vi "Main.vi"() -> ()   [LabVIEW 2021]
doc: "This template is for the Queued Message Handler design pattern.\n\nThe Event Handling Loop generates messages based on user interface actions.\n\nThe Message Handling Loop processes messages generated by the Event Handling Loop, or by other messages. The messages are string values, so new messages can be added easily to the Message Cases case structure in the Message Handling Loop. Each message cluster can also provide an optional value for Message Data, which is a variant that can be converted to whatever message-specific data is required."
uses:
  controls/Air SAS Controls.ctl
  <vilib>/MakerHub/LINX/Private/Type Defs/LINX Ref.ctl
  <vilib>/MakerHub/LINX/Private/Type Defs/Platform.ctl
  <vilib>/MakerHub/LINX/Private/Type Defs/Interface.ctl
  <vilib>/MakerHub/LINX/Private/Device/Type Defs/LINX Device Config.ctl
  <vilib>/MakerHub/LINX/Private/Device/Type Defs/TCP Config.ctl
  <vilib>/MakerHub/LINX/Private/Device/Type Defs/Channels.ctl
  support/Message Queue/Enqueue Message (Single).vi
  <vilib>/MakerHub/LINX/Public/Utilities/Open Serial.vi
  <vilib>/Utility/error.llb/Error Cluster From Error Code.vi
  <vilib>/ErrorRing/Error Ring.xnode
  support/Message Queue/Message Queue.lvlib
  support/User Event - Stop/User Event - Stop.lvlib
  <vilib>/MakerHub/LINX/LMH-LINX.lvlib
  <vilib>/MakerHub/LINX/Private/Device/Device.lvlib
panel:
  in  "Motion Control":bool
  in  "Serial Port":refnum<visa-resource-name>="COM3"
  out "Display <Replace Me>":string
  in  "SAS Data Acquisition":bool
  in  "Waveform Capture":bool
  in  "Exit":bool
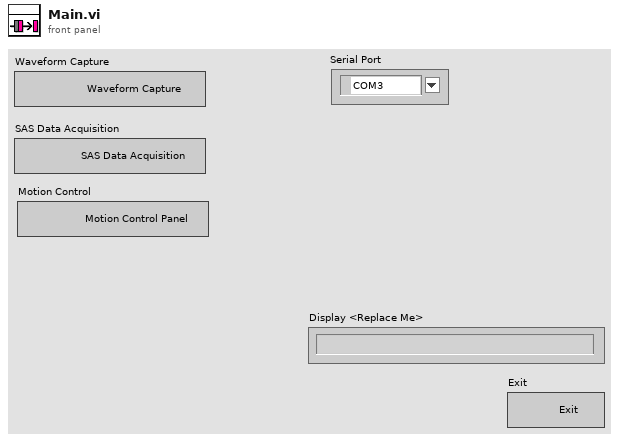
[diagram p1: front panel]
types:
  T1 = enum8{"Enabled", "Disabled", "Disabled and Grayed Out"}
  T2 = typedef "Air SAS Controls.ctl" = cluster{"Receive Duration":dbl, "I/O":cluster{"DAQmx Device":tag, "AO Range":dbl, "AI Range":dbl, "DAQ Group Delay":dbl, "Fs":dbl}, "Hardware":cluster{"Centerpos":dbl[], "TXpos":dbl[], "RX1pos":dbl[], "RX2pos":dbl[], "Angle":dbl, "Height":dbl}, "Waveform":cluster{"LFM Parameters":cluster{"Duration":dbl, "Fstart (Hz)":dbl, "Fstop (Hz)":dbl, "Out. Amplitude (Vpk)":dbl, "Window %":dbl}, "Transmit Waveform":waveform(dbl)}, "LINX Resource":T3, "Port":dbl}
  T3 = typedef "LMH-LINX.lvlib/LINX Ref.ctl" = cluster{"IO":T4, "Interface":T5, "LINX Device Config":T6}
  T4 = typedef "LMH-LINX.lvlib/Platform.ctl" = enum16{"Remote", "Local"}
  T5 = typedef "LMH-LINX.lvlib/Interface.ctl" = enum16{"Serial", "TCP"}
  T6 = typedef "LMH-LINX.lvlib/Device.lvlib/LINX Device Config.ctl" = cluster{"Interface":T5, "COM Port":refnum<visa-resource-name>, "TCP Configuration":T7, "Device Family":u8, "Device ID":u8, "Device Name":string, "TCP Ref":refnum<k5>, "Channels":T8}
  T7 = typedef "LMH-LINX.lvlib/Device.lvlib/TCP Config.ctl" = cluster{"IP Address":string, "Port":u16}
  T8 = typedef "LMH-LINX.lvlib/Channels.ctl" = cluster{"DI":u8[], "DO":u8[], "AI":u8[], "AO":u8[], "PWM":u8[], "QE":u8[], "UART":u8[], "I2C 2":u8[], "SPI":u8[], "CAN":u8[], "Servo":u8[], "AI Ref (V)":dbl, "AI Resolution (Bits)":u8, "AO Ref (V)":dbl, "AO Resolution (Bits)":u8}
  T9 = typedef "Message Queue.lvlib/All Message Queues.ctl" = cluster{"UI":refnum<queue>}
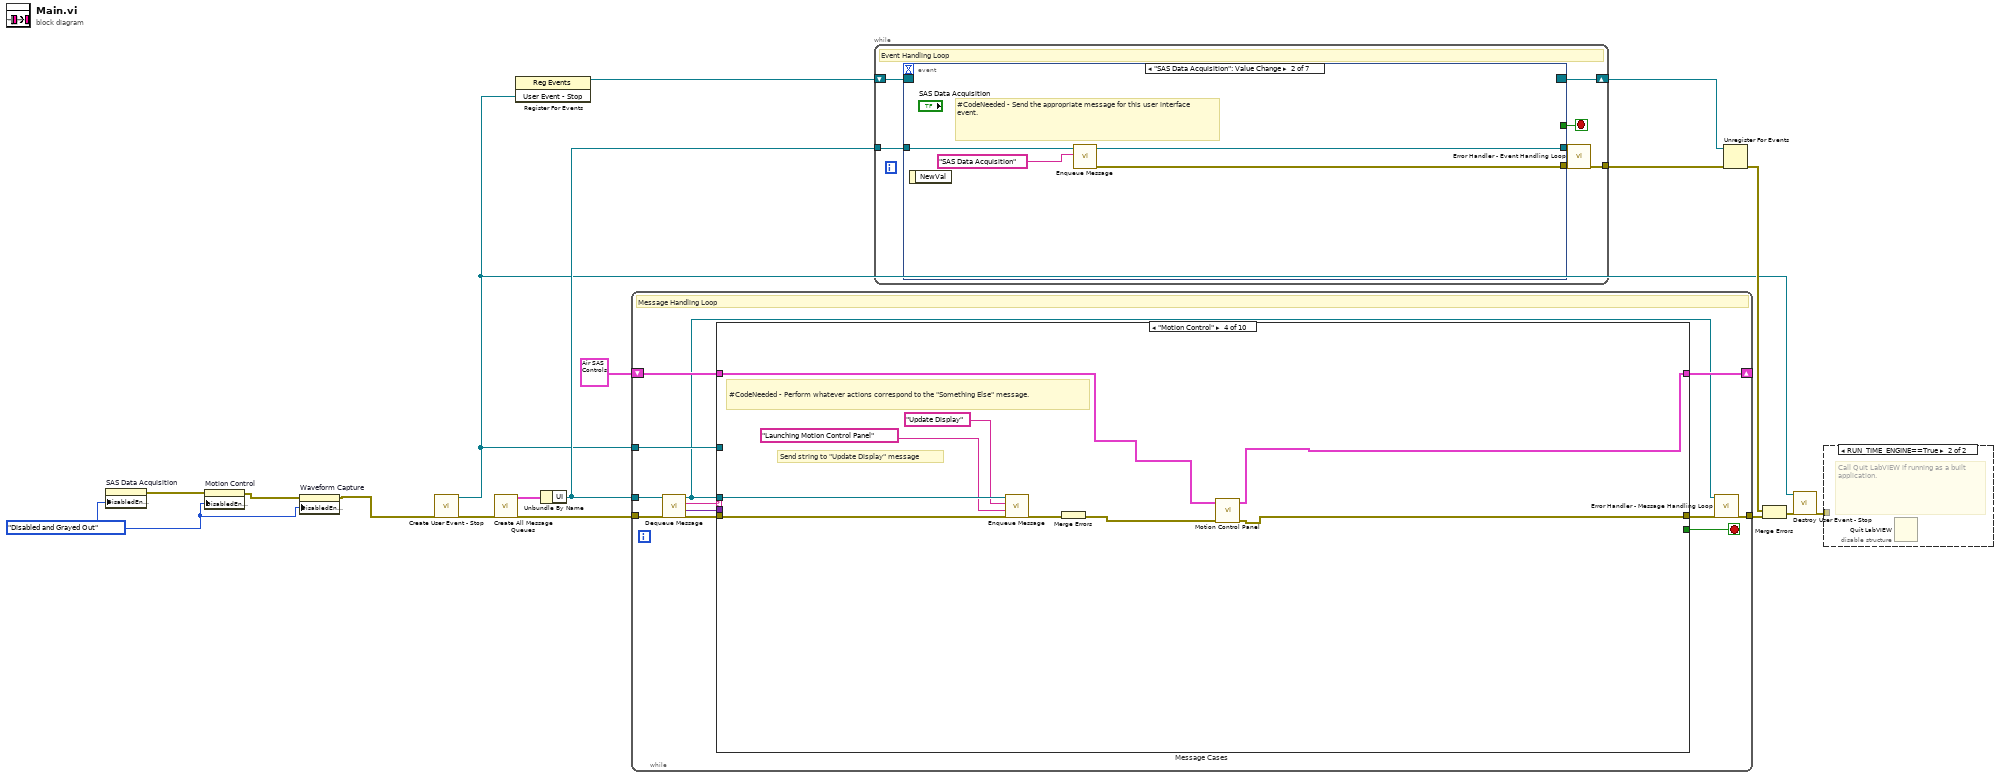
[diagram p0: block diagram]
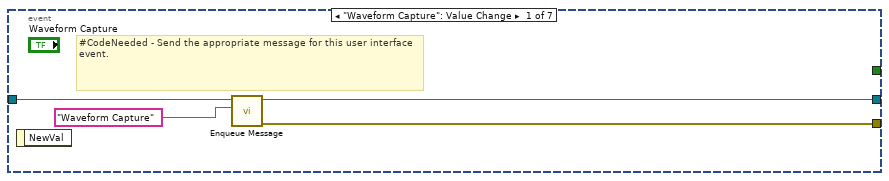
[diagram p3: hidden frame]
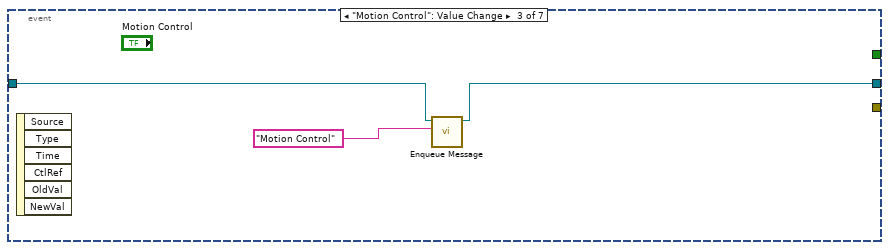
[diagram p4: hidden frame]
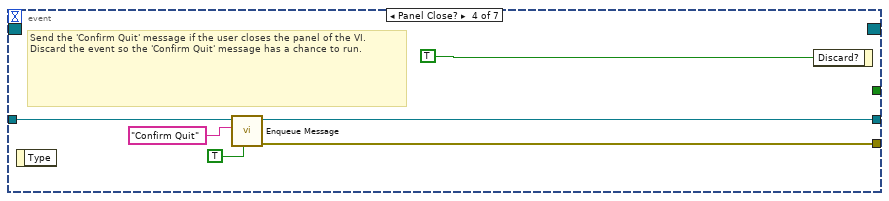
[diagram p5: hidden frame]
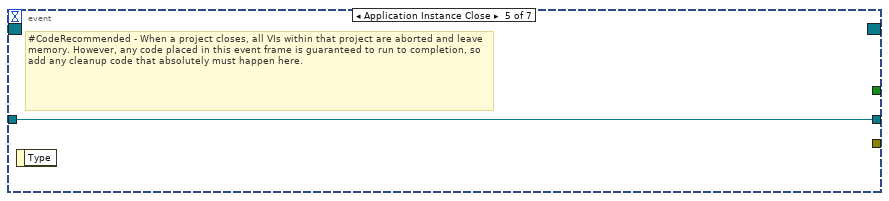
[diagram p6: hidden frame]
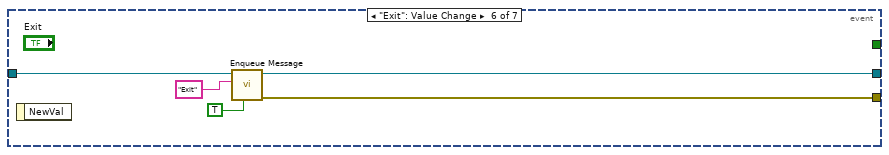
[diagram p7: hidden frame]
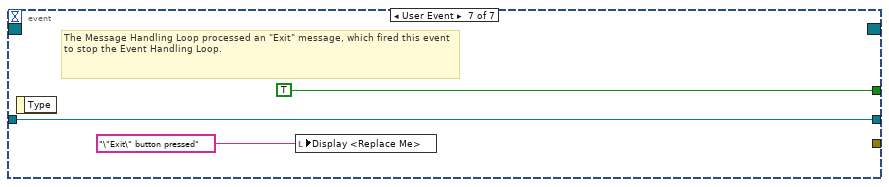
[diagram p8: hidden frame]
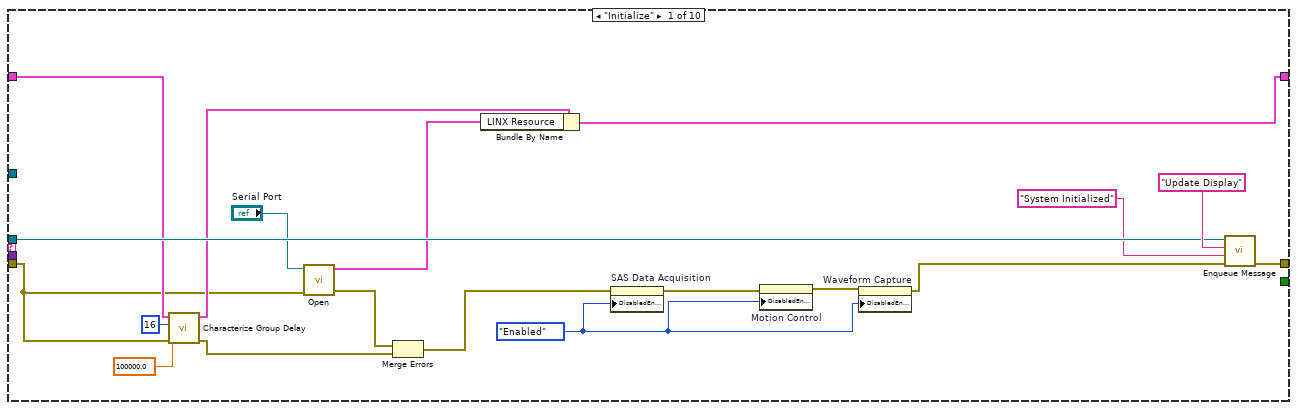
[diagram p9: hidden frame]
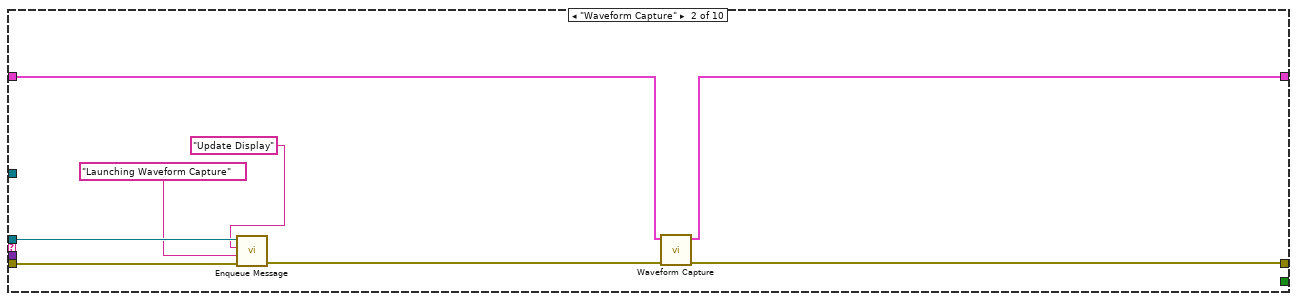
[diagram p10: hidden frame]
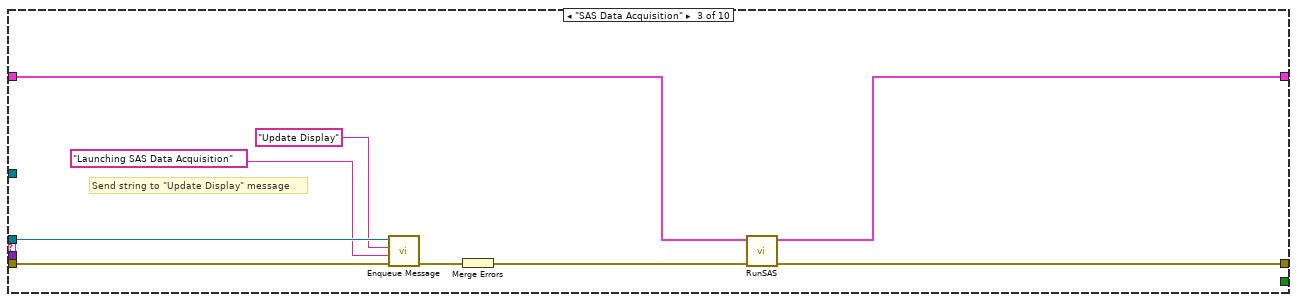
[diagram p11: hidden frame]
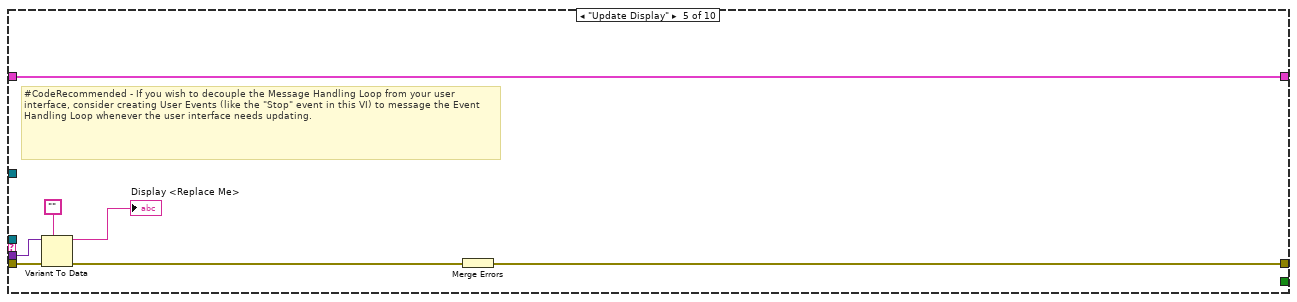
[diagram p12: hidden frame]
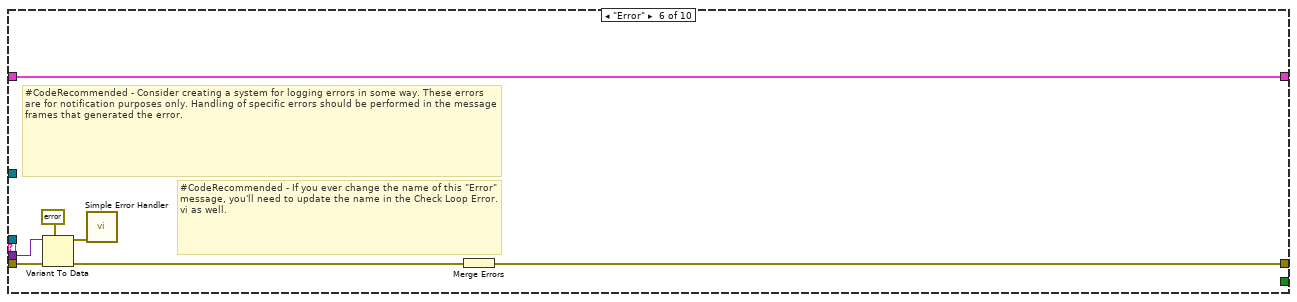
[diagram p13: hidden frame]
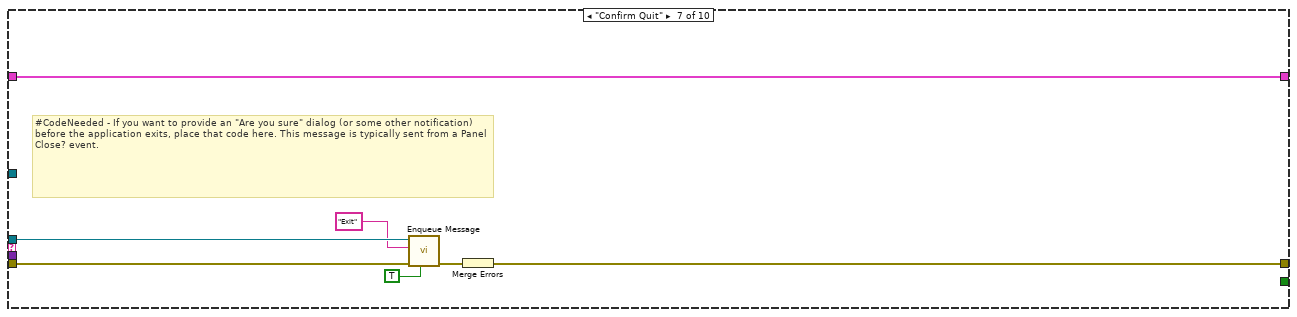
[diagram p14: hidden frame]
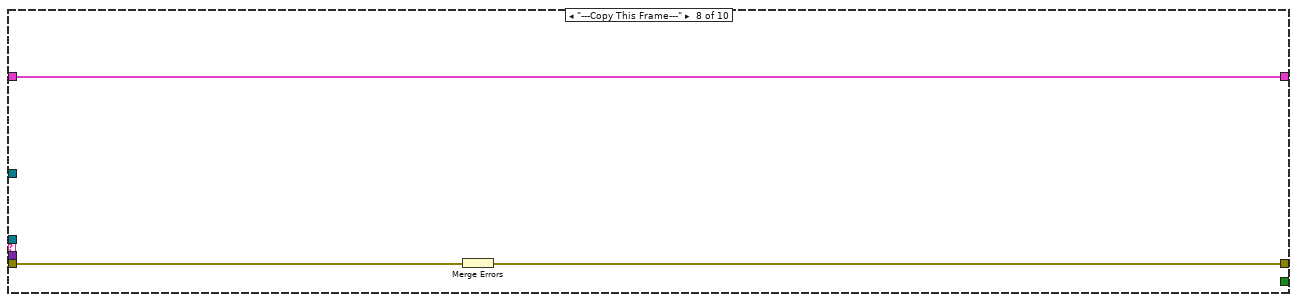
[diagram p15: hidden frame]
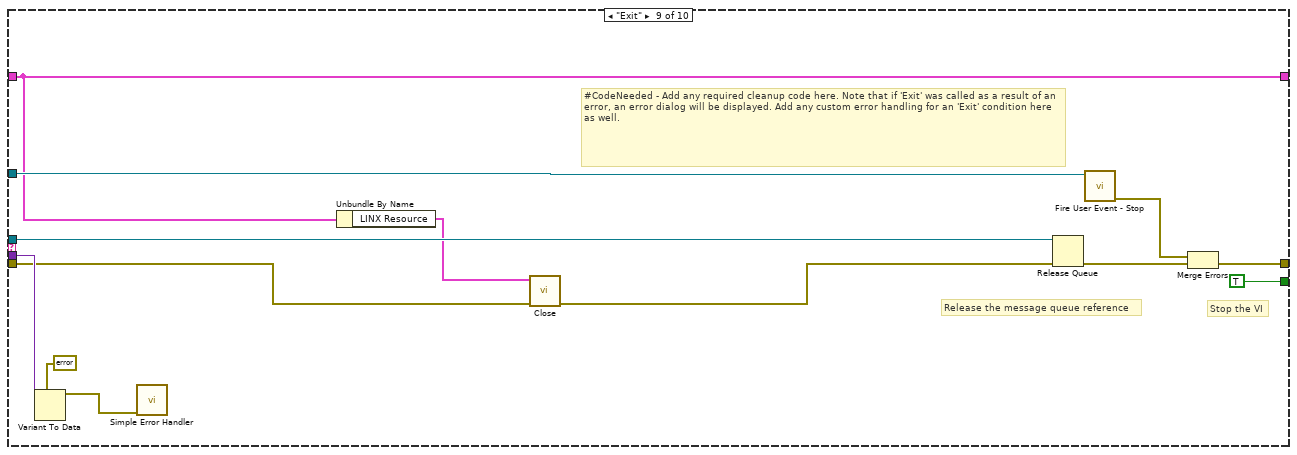
[diagram p16: hidden frame]
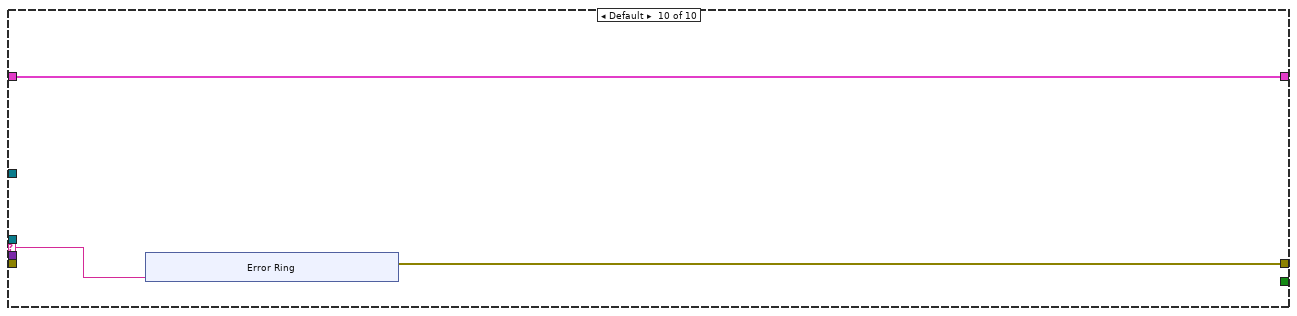
[diagram p17: hidden frame]
diagram:
  w1 = T1."Disabled and Grayed Out" ("Disabled")
  n1 = property on="SAS Data Acquisition" class="Bool"("DisabledEnum"=w1) -> (error out=w4:errorcluster)  [unwired: 2 in, 1 out]
  n2 = property on="Motion Control" class="Bool"(error in=w4, "DisabledEnum"=w1) -> (error out=w3:errorcluster)  [unwired: 1 in, 1 out]
  n3 = property on="Waveform Capture" class="Bool"(error in=w3, "DisabledEnum"=w1) -> (error out=w2:errorcluster)  [unwired: 1 in, 1 out]
  n4 = call "Create User Event - Stop.vi"("error in (no error)"=w2) -> ("error out"=w13:errorcluster, "User Event - Stop"=w6:refnum<user-event>)  [unwired: 9 in]
  n5 = call "Create All Message Queues.vi"("error in (no error)"=w13) -> ("error out"=w17:errorcluster, "Message Queues out"=w16:T9)  [unwired: 9 in]
  n6 = register-events(w6) -> (reference out=w7:refnum<event-registration>)  [unwired: 2 in, 1 out]
  n7 = Unbundle By Name(w16) -> ("UI"=w14:refnum<queue>)
  n8 = while {
    tunnel: w14 -> [w21]
    shift-right: [w28] -> _
    shift-left: T2 {"Receive Duration"=0.0, "I/O"={"DAQmx Device"="Dev1", "AO Range"=0.0, "AI Range"=0.0, "DAQ Group Delay"=0.0, "Fs"=0.0}, "Hardware"={"Centerpos"=[0.0, 0.0, 0.0], "TXpos"=[0.0, 0.0, 0.0], "RX1pos"=[0.0, 0.0, 0.0], "RX2pos"=[0.0, 0.0, 0.0], "Angle"=0.0, "Height"=0.0}, "Waveform"={"LFM Parameters"={"Duration"=1.0, "Fstart (Hz)"=1000.0, "Fstop (Hz)"=10000.0, "Out. Amplitude (Vpk)"=1.0, "Window %"=10.0}, "Transmit Waveform"={"t0"=timestamp(0 s since 1904-01-01), "dt"=1.0, "Y"=[]}}, "LINX Resource"={"IO"=enum."Remote", "Interface"=enum."Serial", "LINX Device Config"={"Interface"=enum."Serial", "COM Port"="COM13", "TCP Configuration"={"IP Address"="", "Port"=0}, "Device Family"=1, "Device ID"=1, "Device Name"="myRIO-1900", "TCP Ref"=refnum, "Channels"={"DI"=[0, 1, 2, 3, 4, 5, 6, 7, 8, 9, 10, 11, 12, 13, 14, 15, 16, 17, 18, 19, 20, 21, 22, 23, 24, 25, 26, 27, 28, 29, 30, 31, 32, 33, 34, 35, 36, 37, 38, 39, 40, 41, 42, 43, 44, 45, 46], "DO"=[0, 1, 2, 3, 4, 5, 6, 7, 8, 9, 10, 11, 12, 13, 14, 15, 16, 17, 18, 19, 20, 21, 22, 23, 24, 25, 26, 27, 28, 29, 30, 31, 32, 33, 34, 35, 36, 37, 38, 39, 40, 41, 42, 43, 44, 45, 46], "AI"=[0, 1, 2, 3, 4, 5, 6, 7, 8, 9, 10, 11], "AO"=[], "PWM"=[3, 5, 6, 9, 10], "QE"=[], "UART"=[0, 1], "I2C 2"=[0], "SPI"=[0], "CAN"=[], "Servo"=[], "AI Ref (V)"=0.0, "AI Resolution (Bits)"=0, "AO Ref (V)"=0.0, "AO Resolution (Bits)"=0}}}, "Port"=3000.0} ("AirSAS Controls") -> [w29]
    tunnel: w6 -> [w26]
    tunnel: w17 -> [w25]
    tunnel: [w19] -> w15
    stop <- w27 stop-if-true
    # "Message Handling Loop"
    n9 = call "Dequeue Message.vi"("error in (no error)"=w25, "Message Queue"=w21) -> ("error out"=w24:errorcluster, "Message Data"=w22:variant, "Message"=w23:string, "dup Message Queue"=w20:refnum<queue>)  [unwired: 6 in]
    n10 = case "Message Cases" shown="\"Motion Control\"" w23 {
      selector: w23 -> [_ _ _ _ _ _ _ _ _ w112]
      tunnel: w20 -> [w46 w55 w63 w72 _ _ w91 _ w111 _]
      tunnel: w24 -> [w33 w56 w65 w74 w79 w88 w95 w98 w102 _]
      tunnel: [w48 w51 w59 w69 w80 w82 w93 w96 w108 w113] -> w18
      tunnel: w29 -> [w35 w50 w57 w68 w81 w87 w94 w97 w100 w114]
      tunnel: [w43 w49 w58 w67 w81 w87 w94 w97 w100 w114] -> w28
      tunnel: [_ _ _ _ _ _ _ _ TRUE _] -> w27
      tunnel: w22 -> [_ _ _ _ w78 w86 _ _ w103 _]
      tunnel: w26 -> [_ _ _ _ _ _ _ _ w107 _]
      frame "Initialize" {
        w36 = T1."Enabled" ("Disabled")
        # "Initialize - All initialization work should take place in this message, since other loops can potentially enqueue messages that execute immediately after this one."
        n11 = call "Characterize Group Delay.vi"("error in (no error)"=w33, "sample frequency [Hz]"=100000.0, "number of averages"=16, "AirSAS Controls Out"=w35) -> ("error out"=w32:errorcluster, "AirSAS Controls Out"=w34:T2)  [unwired: 6 in]
        n12 = call-poly <vilib>:"Open.vi"("Error In"=w33, "Serial Port"="Serial Port") -> ("Error Out"=w40:errorcluster, "LINX Resource"=w42:T3)  [unwired: 7 in, 1 out]
        n13 = Merge Errors(w40, w32) -> (w39:errorcluster)
        n14 = Bundle By Name(cluster=w34, "LINX Resource"=w42) -> (w43:T2)
        n15 = property on="SAS Data Acquisition" class="Bool"(error in=w39, "DisabledEnum"=w36) -> (error out=w41:errorcluster)  [unwired: 1 in, 1 out]
        n16 = property on="Motion Control" class="Bool"(error in=w41, "DisabledEnum"=w36) -> (error out=w38:errorcluster)  [unwired: 1 in, 1 out]
        n17 = property on="Waveform Capture" class="Bool"(error in=w38, "DisabledEnum"=w36) -> (error out=w37:errorcluster)  [unwired: 1 in, 1 out]
        n18 = call-poly "Enqueue Message.vi"("error in (no error)"=w37, "Message Data"="System Initialized" ("Initial Message"), "Message"="Update Display", "Message Queue"=w46) -> ("error out"=w48:errorcluster)  [unwired: 6 in, 1 out]
      }
      frame "Waveform Capture" {
        # "Something - Replace this message with functionality for your own application."
        n19 = call-poly "Enqueue Message.vi"("error in (no error)"=w56, "Message Data"="Launching Waveform Capture" ("\"Do Something\" button pressed"), "Message"="Update Display", "Message Queue"=w55) -> ("error out"=w52:errorcluster)  [unwired: 6 in, 1 out]
        n20 = call "Waveform Capture.vi"("error in (no error)"=w52, "AirSAS Controls"=w50) -> ("error in (no error) 2"=w51:errorcluster, "AirSAS Controls 2"=w49:T2)  [unwired: 8 in]
      }
      frame "SAS Data Acquisition" {
        # "Send string to \"Update Display\" message"
        # "Something Else - Replace this message with functionality for your own application."
        n21 = call-poly "Enqueue Message.vi"("error in (no error)"=w65, "Message Data"="Launching SAS Data Acquisition" ("\"Do Something Else\" button pressed"), "Message"="Update Display", "Message Queue"=w63) -> ("error out"=w64:errorcluster)  [unwired: 6 in, 1 out]
        n22 = Merge Errors(w64) -> (w60:errorcluster)
        n23 = call "RunSAS.vi"("error in"=w60, "AirSAS Controls"=w57) -> ("error out"=w59:errorcluster, "AirSAS Controls 2"=w58:T2)  [unwired: 8 in]
      }
      frame "Motion Control" {
        # "Send string to \"Update Display\" message"
        # "#CodeNeeded - Perform whatever actions correspond to the \"Something Else\" message."
        # "Something Else - Replace this message with functionality for your own application."
        n24 = call-poly "Enqueue Message.vi"("error in (no error)"=w74, "Message Data"="Launching Motion Control Panel" ("\"Do Something Else\" button pressed"), "Message"="Update Display", "Message Queue"=w72) -> ("error out"=w73:errorcluster)  [unwired: 6 in, 1 out]
        n25 = Merge Errors(w73) -> (w66:errorcluster)
        n26 = call "Motion Control Panel.vi"("Error Out"=w66, "AirSAS Controls"=w68) -> ("Error Out 2"=w69:errorcluster, "output cluster"=w67:T2)  [unwired: 8 in]
      }
      frame "Update Display" {
        # "#CodeRecommended - If you wish to decouple the Message Handling Loop from your user interface, consider creating User Events (like the \"Stop\" event in this VI) to message the Event Handling Loop whenever the user interface needs updating."
        # "Update Display - Convert the message data to a string to display in the Data Display indicator."
        n27 = Variant To Data(error in=w79, type="", Variant=w78) -> (data=→"Display <Replace Me>":string, error out=w76:errorcluster)
        n28 = Merge Errors(w76) -> (w80:errorcluster)
      }
      frame "Error" {
        # "#CodeRecommended - If you ever change the name of this \"Error\" message, you'll need to update the name in the Check Loop Error.vi as well."
        # "#CodeRecommended - Consider creating a system for logging errors in some way. These errors are for notification purposes only. Handling of specific errors should be performed in the message frames that generated the error."
        # "Error - Display an error dialog. This message is sent by the \"Error Handler\" VIs at the end of other loops in this application."
        n29 = Variant To Data(error in=w88, type=errorcluster {"status"=FALSE, "code"=0, "source"=""} ("error constant"), Variant=w86) -> (data=w84:errorcluster, error out=w83:errorcluster)
        n30 = call <vilib>:"Simple Error Handler.vi"("error in (no error)"=w84) -> ()  [unwired: 4 in, 5 out]
        n31 = Merge Errors(w83) -> (w82:errorcluster)
      }
      frame "Confirm Quit" {
        # "#CodeNeeded - If you want to provide an \"Are you sure\" dialog (or some other notification) before the application exits, place that code here. This message is typically sent from a Panel Close? event."
        # "Confirm Quit - Message that can confirm whether or not the user wants to exit the application."
        n32 = call-poly "Enqueue Message.vi"("Priority Message? (F)"=TRUE, "error in (no error)"=w95, "Message"="Exit", "Message Queue"=w91) -> ("error out"=w92:errorcluster)  [unwired: 6 in, 1 out]
        n33 = Merge Errors(w92) -> (w93:errorcluster)
      }
      frame "---Copy This Frame---" {
        # "Duplicate this frame when creating new messages.  Change this comment in the duplicated frame to describe this message."
        n34 = Merge Errors(w98) -> (w96:errorcluster)
      }
      frame "Exit" {
        # "Stop the VI"
        # "Release the message queue reference"
        # "#CodeNeeded - Add any required cleanup code here. Note that if 'Exit' was called as a result of an error, an error dialog will be displayed. Add any custom error handling for an 'Exit' condition here as well."
        n35 = Variant To Data(type=errorcluster {"status"=FALSE, "code"=0, "source"=""} ("error constant"), Variant=w103) -> (data=w104:errorcluster)  [unwired: 1 in, 1 out]
        n36 = call <vilib>:"Simple Error Handler.vi"("error in (no error)"=w104) -> ()  [unwired: 4 in, 5 out]
        n37 = Unbundle By Name(w100) -> ("LINX Resource"=w99:T3)
        n38 = call <vilib>:"Close.vi"("Error In"=w102, "LINX Resource"=w99) -> ("Error Out"=w101:errorcluster)  [unwired: 9 in]
        n39 = Release Queue(queue=w111, error in (no error)=w101) -> (error out=w109:errorcluster)  [unwired: 1 in, 2 out]
        n40 = call "Fire User Event - Stop.vi"("User Event - Stop"=w107) -> ("error out"=w106:errorcluster)  [unwired: 10 in]
        n41 = Merge Errors(w106, w109) -> (w108:errorcluster)
      }
      frame Default {
        # "'Default' case only runs if there is a message that isn't defined in any of the other cases.  Output a programming error."
        n42 = xnode "Error Ring"("parameter 0"=w112) -> ("error out"=w113:errorcluster)
      }
    }
    n43 = call "Error Handler - Message Handling Loop.vi"("error in (no error)"=w18, "Message Queue"=w20) -> ("dup error in"=w19:errorcluster)  [unwired: 8 in, 1 out]
  }
  n44 = while {
    tunnel: w14 -> [w128]
    shift-right: [w126] -> w10
    shift-left: w7 -> [w127]
    tunnel: [w122] -> w8
    stop <- w124 stop-if-true
    # "Event Handling Loop"
    n45 = event shown="[1] \"SAS Data Acquisition\": Value Change" {
      selector: w127 -> [_ _ _ _ _ _ _]
      dyn-events: [_ _ _ _ _ _ _] -> w126
      timeout: _ -> [_ _ _ _ _ _ _]
      tunnel: [_ _ _ _ _ _ TRUE ("Discard?")] -> w124
      tunnel: w128 -> [w132 w136 w138 w144 w146 w151 w154]
      tunnel: [w129 w133 _ w143 _ w150 _] -> w125
      tunnel: [w131 w135 w137 w142 w146 w149 w154] -> w123
      event "Waveform Capture": Value Change {
        # "#CodeNeeded - Send the appropriate message for this user interface event."
        n46 = event-data() -> ()  [unwired: 1 in, 1 out]
        n47 = call-poly "Enqueue Message.vi"("Message"="Waveform Capture", "Message Queue"=w132) -> ("error out"=w129:errorcluster, "dup Message Queue"=w131:refnum<queue>)  [unwired: 8 in]
      }
      event "SAS Data Acquisition": Value Change {
        # "#CodeNeeded - Send the appropriate message for this user interface event."
        n48 = event-data() -> ()  [unwired: 1 in, 1 out]
        n49 = call-poly "Enqueue Message.vi"("Message"="SAS Data Acquisition", "Message Queue"=w136) -> ("error out"=w133:errorcluster, "dup Message Queue"=w135:refnum<queue>)  [unwired: 8 in]
      }
      event "Motion Control": Value Change {
        n50 = event-data() -> ()  [unwired: 1 in, 6 out]
        n51 = call-poly "Enqueue Message.vi"("Message"="Motion Control", "Message Queue"=w138) -> ("dup Message Queue"=w137:refnum<queue>)  [unwired: 8 in, 1 out]
      }
      event Panel Close? {
        # "Send the 'Confirm Quit' message if the user closes the panel of the VI. Discard the event so the 'Confirm Quit' message has a chance to run."
        n52 = event-data() -> ()  [unwired: 1 in, 1 out]
        n53 = call-poly "Enqueue Message.vi"("Priority Message? (F)"=TRUE, "Message"="Confirm Quit", "Message Queue"=w144) -> ("error out"=w143:errorcluster, "dup Message Queue"=w142:refnum<queue>)  [unwired: 7 in]
        n54 = event-data("Discard?"=TRUE) -> ()  [unwired: 1 in, 1 out]
      }
      event Application Instance Close {
        # "#CodeRecommended - When a project closes, all VIs within that project are aborted and leave memory. However, any code placed in this event frame is guaranteed to run to completion, so add any cleanup code that absolutely must happen here."
        n55 = event-data() -> ()  [unwired: 1 in, 1 out]
      }
      event "Exit": Value Change {
        n56 = event-data() -> ()  [unwired: 1 in, 1 out]
        n57 = call-poly "Enqueue Message.vi"("Priority Message? (F)"=TRUE, "Message"="Exit", "Message Queue"=w151) -> ("error out"=w150:errorcluster, "dup Message Queue"=w149:refnum<queue>)  [unwired: 7 in]
      }
      event User Event {
        # "The Message Handling Loop processed an \"Exit\" message, which fired this event to stop the Event Handling Loop."
        n58 = event-data() -> ()  [unwired: 1 in, 1 out]
        n59 = local write "Display <Replace Me>"("\"Exit\" button pressed" ("VI Stopped")) -> ()
      }
    }
    n60 = call "Error Handler - Event Handling Loop.vi"("error in (no error)"=w125, "Message Queue"=w123) -> ("dup error in"=w122:errorcluster)  [unwired: 8 in, 1 out]
  }
  n61 = Unregister For Events(event registration refnum=w10, error in=w8) -> (error out=w11:errorcluster)
  n62 = Merge Errors(w11, w15) -> (w12:errorcluster)
  n63 = call "Destroy User Event - Stop.vi"("error in (no error)"=w12, "User Event - Stop"=w6) -> ("error out"=w9:errorcluster)  [unwired: 9 in]
  n64 = disable-structure shown="RUN_TIME_ENGINE==True" {
    disable-tunnel: w9 -> [_ _]
    frame condition #0 (active) {
    }
    frame condition #1 {
      # "Call Quit LabVIEW if running as a built application."
      n65 = Quit LabVIEW() -> ()  [unwired: 1 in]
    }
  }
